vi "fastseq_set_fastChannel.vi"(8 "pan-channel":T1 {"channel" max=7 step=1; "panel" max=7 step=1}, 9 "is dummy?":bool, 10 "fast chan number":u8, 11 "FPGA VI Reference In":T2) -> (3 "FPGA VI Reference Out":T2)   [LabVIEW 2013]
uses:
  fpga-bitfile-ref.ctl
  DAC/backend/typedefs/panel-channel.ctl
  slot-use-type.ctl
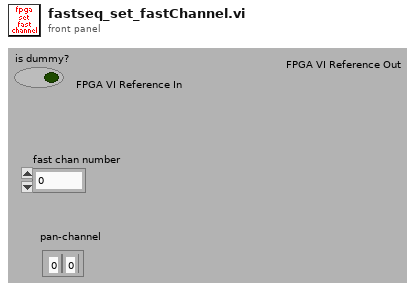
[diagram p1: front panel]
types:
  T1 = typedef "panel-channel.ctl" = cluster{"panel":u8, "channel":u8}
  T2 = typedef "fpga-bitfile-ref.ctl" = refnum<k20>
  T3 = typedef "slot-use-type.ctl" = fxp<+,4,4>
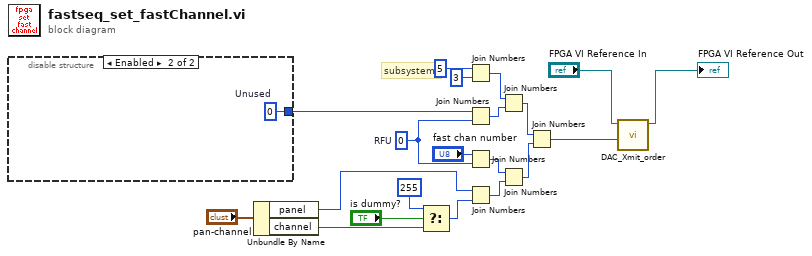
[diagram p0: block diagram]
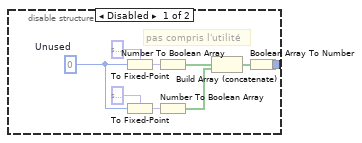
[diagram p2: hidden frame]
diagram:
  w7 = u8 0  # RFU
  # "subsystem"
  n1 = disable-structure shown="Enabled" {
    disable-tunnel: [w22 w30] -> w11
    frame Disabled {
      w21 = u8 0  # Unused
      # "pas compris l'utilité"
      n2 = To Fixed-Point(fixed-point type=T3 0.0, number=w21) -> (fixed-point=w26:T3)
      n3 = To Fixed-Point(fixed-point type=T3 0.0, number=w21) -> (fixed-point=w25:T3)
      n4 = Number To Boolean Array(number=w26) -> (Boolean array=w27:bool[])
      n5 = Number To Boolean Array(number=w25) -> (Boolean array=w29:bool[])
      n6 = Build Array (concatenate)(w27, w29) -> (w28:bool[])
      n7 = Boolean Array To Number(Boolean array=w28) -> (number=w22:u8)
    }
    frame Enabled {
      w30 = u8 0  # Unused
    }
  }
  n8 = Unbundle By Name("pan-channel") -> ("panel"=w1:u8, "channel"=w4:u8)
  n9 = Select(t=u8 255, s="is dummy?", f=w4) -> (s? t:f=w5:u8)
  n10 = Join Numbers(hi=u8 5, lo=u8 3) -> ((hi.lo)=w16:u16)
  n11 = Join Numbers(hi=w11, lo=w7) -> ((hi.lo)=w17:u16)
  n12 = Join Numbers(hi="fast chan number", lo=w7) -> ((hi.lo)=w8:u16)
  n13 = Join Numbers(hi=w1, lo=w5) -> ((hi.lo)=w9:u16)
  n14 = Join Numbers(hi=w16, lo=w17) -> ((hi.lo)=w13:u32)
  n15 = Join Numbers(hi=w8, lo=w9) -> ((hi.lo)=w14:u32)
  n16 = Join Numbers(hi=w13, lo=w14) -> ((hi.lo)=w20:u64)
  n17 = call "DAC_Xmit_order.vi"("Order in"=w20, "FPGA VI Reference In"="FPGA VI Reference In") -> ("FPGA VI Reference Out"=→"FPGA VI Reference Out":T2)  [unwired: 9 out]
